vi "Facade.vi"(0 "Data In":T4 {"time" format="%<%H:%M:%S>T"}, 2 "Display State In":T2 {"time" format="%<%.3X>T"}, 3 "Container State":T3) -> (6 "Data Out":T4 {"time" format="%<%H:%M:%S>T"}, 7 "Display State Out":T2 {"time" format="%<%.3X>T"}, 8 "Action":T1)   [LabVIEW 2013, in "Altitude2.xctl"]
uses:
  Altitude2.xctl
  Data.ctl
  <vilib>/_xctls/Container State.ctl
  State ctl.ctl
  <vilib>/_xctls/Action.ctl
  <vilib>/_xctls/XControlSupport.lvlib
panel:
  out "altitude":cluster{timestamp[], dbl[]}(graph)
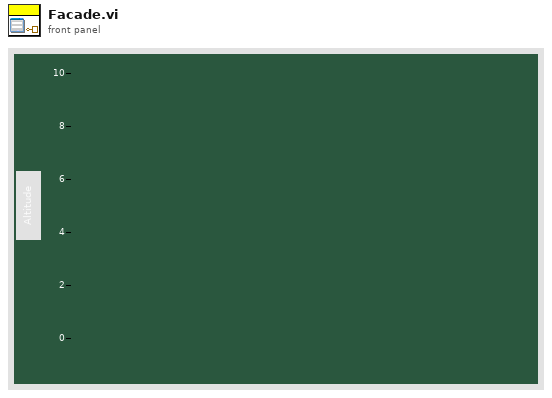
[diagram p1: front panel]
types:
  T1 = typedef "XControlSupport.lvlib/Action.ctl" = cluster{"Data Changed?":bool, "State Changed?":bool, "Action Name":string}
  T2 = typedef "Altitude2.xctl/State ctl.ctl" = cluster{"time":timestamp[], "altitude":dbl[]}
  T3 = typedef "XControlSupport.lvlib/Container State.ctl" = cluster{"Indicator?":bool, "Run Mode?":bool, " Refnum":refnum<vi>}
  T4 = typedef "Altitude2.xctl/Data.ctl" = cluster{"time":timestamp, "altitude":dbl}
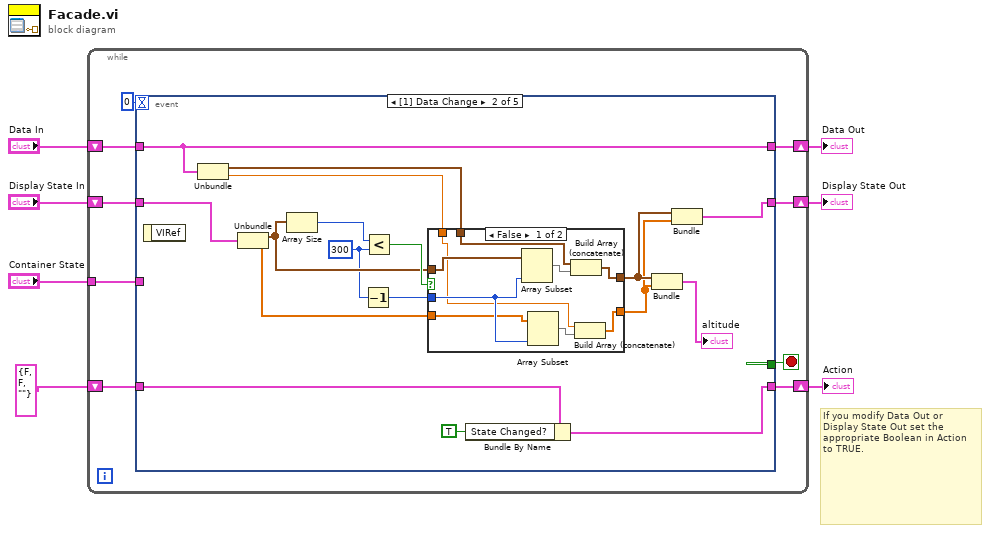
[diagram p0: block diagram]
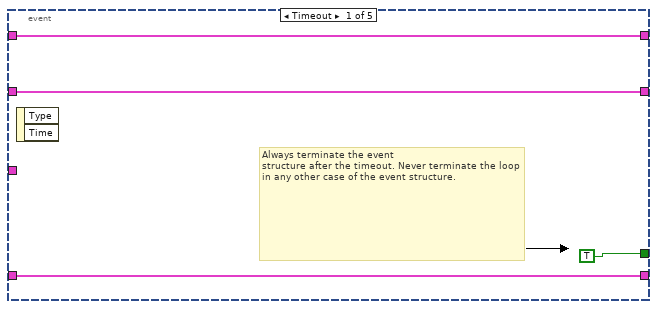
[diagram p2: hidden frame]
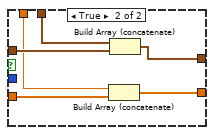
[diagram p3: hidden frame]
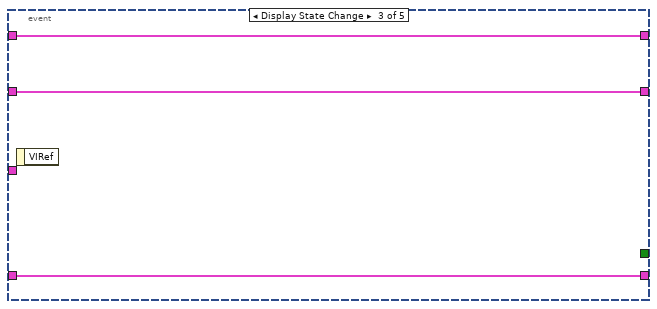
[diagram p4: hidden frame]
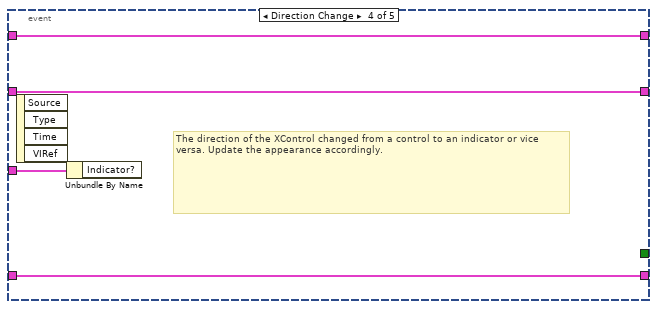
[diagram p5: hidden frame]
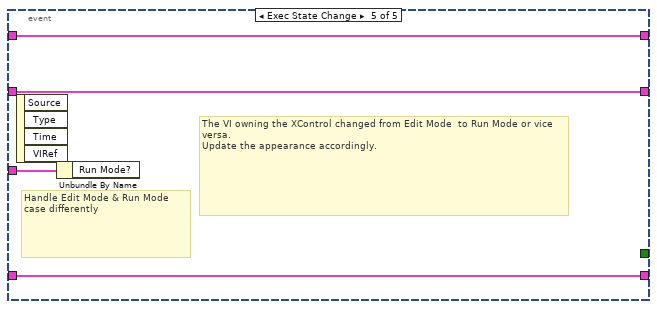
[diagram p6: hidden frame]
diagram:
  # "If you modify Data Out or\nDisplay State Out set the\nappropriate Boolean in Action\nto TRUE."
  n1 = while {
    shift-right: [w15] -> w4
    shift-left: "Display State In" -> [w16]
    tunnel: "Container State" -> [w12]
    shift-right: [w10] -> w7
    shift-left: "Data In" -> [w11]
    shift-right: [w8] -> w2
    shift-left: T1 {"Data Changed?"=FALSE, "State Changed?"=FALSE, "Action Name"=""} ("Action") -> [w9]
    stop <- w14 stop-if-true
    n2 = event shown="[1] Data Change" {
      selector: _ -> [_ _ _ _ _]
      dyn-events: _ -> [_ _ _ _ _]
      timeout: 0 -> [_ _ _ _ _]
      tunnel: w16 -> [w18 w37 w55 w58 w62]
      tunnel: [w18 w21 w55 w58 w62] -> w15
      tunnel: [TRUE _ _ _ _] -> w14
      tunnel: w12 -> [_ _ _ w59 w63]
      tunnel: w11 -> [w17 w34 w54 w57 w61]
      tunnel: [w17 w34 w54 w57 w61] -> w10
      tunnel: [w19 w24 w53 w56 w60] -> w8
      tunnel: w9 -> [w19 w26 w53 w56 w60]
      event Timeout {
        # "Always terminate the event\nstructure after the timeout. Never terminate the loop in any other case of the event structure."
        n3 = event-data() -> ()  [unwired: 1 in, 2 out]
      }
      event Data Change {
        w28 = 300 ("y")
        n4 = event-data() -> ()  [unwired: 1 in, 1 out]
        n5 = Unbundle(w34) -> ("time"=w33:timestamp, "altitude"=w32:dbl)
        n6 = Unbundle(w37) -> ("time"=w31:timestamp[], "altitude"=w30:dbl[])
        n7 = Array Size(array=w31) -> (size(s)=w36:i32)
        n8 = Decrement(x=w28) -> (x-1=w27:i32)
        n9 = Less?(x=w36, y=w28) -> (x < y?=w35:bool)
        n10 = case shown="False" w35 {
          tunnel: w33 -> [w44 w52]
          tunnel: w32 -> [w39 w50]
          tunnel: w31 -> [w46 w51]
          tunnel: w30 -> [w41 w49]
          tunnel: [w43 w48] -> w23
          tunnel: [w38 w47] -> w22
          tunnel: w27 -> [w42 _]
          frame False {
            n11 = Array Subset(array=w46, length=w42) -> (w45:timestamp[])  [unwired: 1 in]
            n12 = Array Subset(array=w41, length=w42) -> (w40:dbl[])  [unwired: 1 in]
            n13 = Build Array (concatenate)(w44, w45) -> (w43:timestamp[])
            n14 = Build Array (concatenate)(w39, w40) -> (w38:dbl[])
          }
          frame True {
            n15 = Build Array (concatenate)(w50, w49) -> (w47:dbl[])
            n16 = Build Array (concatenate)(w52, w51) -> (w48:timestamp[])
          }
        }
        n17 = Bundle By Name(cluster=w26, "State Changed?"=TRUE) -> (w24:T1)
        n18 = Bundle(w23, w22) -> (→"altitude":cluster{timestamp[], dbl[]})  [unwired: 1 in]
        n19 = Bundle(w23, w22) -> (w21:cluster{timestamp[], dbl[]})  [unwired: 1 in]
      }
      event Display State Change {
        n20 = event-data() -> ()  [unwired: 1 in, 1 out]
      }
      event Direction Change {
        # "The direction of the XControl changed from a control to an indicator or vice versa. Update the appearance accordingly."
        n21 = event-data() -> ()  [unwired: 1 in, 4 out]
        n22 = Unbundle By Name(w59) -> ()  [unwired: 1 out]
      }
      event Exec State Change {
        # "The VI owning the XControl changed from Edit Mode  to Run Mode or vice versa.\nUpdate the appearance accordingly."
        # "Handle Edit Mode & Run Mode\ncase differently"
        n23 = event-data() -> ()  [unwired: 1 in, 4 out]
        n24 = Unbundle By Name(w63) -> ()  [unwired: 1 out]
      }
    }
  }
  "Display State Out" <- w4
  "Data Out" <- w7
  "Action" <- w2
